vi "Arrow Drawing Utility.vi"(0 "LF Pod Setpoint":cluster{"Velocity":dbl, "Theta":dbl}, 5 "LB Pod Setpoint":cluster{"Velocity":dbl, "Theta":dbl}, 7 "RF Pod Setpoint":cluster{"Velocity":dbl, "Theta":dbl}, 9 "RB Pod Setpoint":cluster{"Velocity":dbl, "Theta":dbl}, 12 "cross products":T1, 13 "Translation":dbl[](array[numeric])) -> (4 "Pod Vectors":cluster{dbl[], dbl[]}[](array[cluster]), 6 "Translation Vectors":cluster{dbl[], dbl[]}, 8 "Rotation Vectors":cluster{dbl[], dbl[]})   [LabVIEW 2020]
uses:
  <vilib>/ptbypt/NI_PtbyPt.lvlib
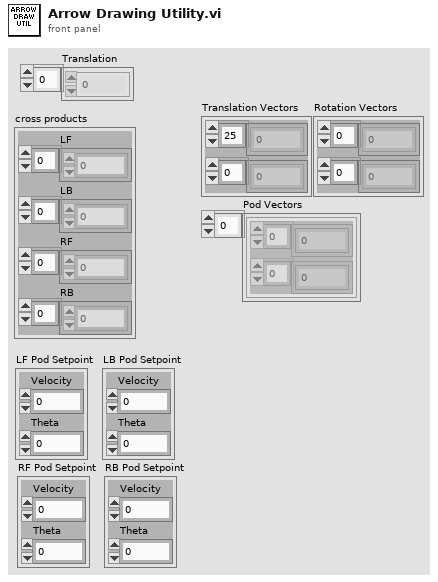
[diagram p1: front panel]
types:
  T1 = cluster{"LF":dbl[], "LB":dbl[], "RF":dbl[], "RB":dbl[]}
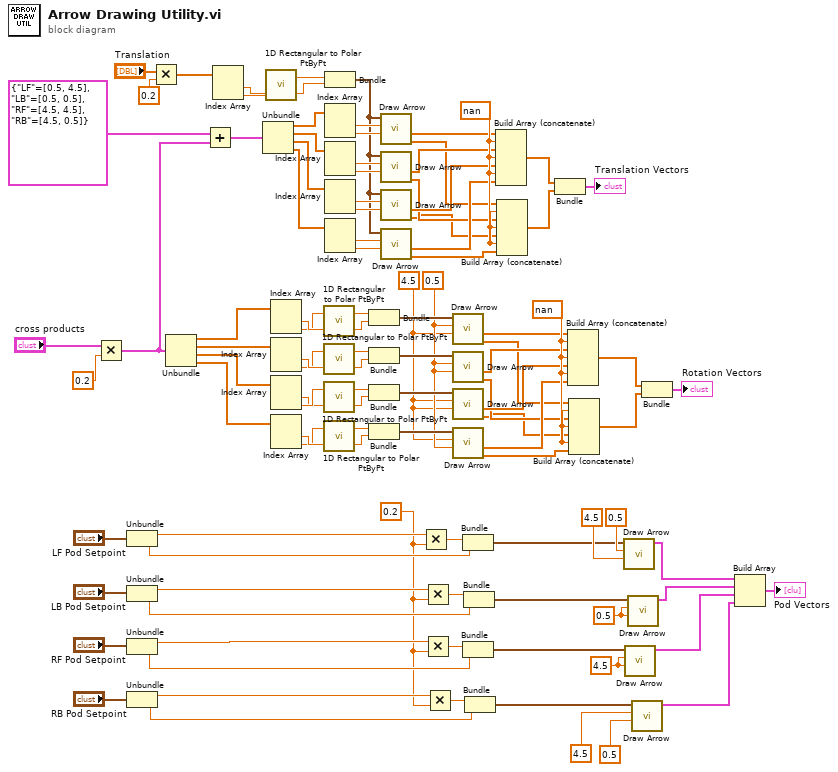
[diagram p0: block diagram]
diagram:
  w41 = nan ("Start Y")
  w54 = nan ("Start Y")
  w55 = 4.5 ("Start Y")
  w56 = 0.5 ("Start X")
  w81 = 0.2 ("y")
  w106 = 4.5 ("Start X")
  w107 = 0.5 ("Start X")
  n1 = Multiply(x="cross products", y=0.2) -> (x*y=w7:T1)
  n2 = Unbundle("LF Pod Setpoint") -> ("Velocity"=w97:dbl, "Theta"=w92:dbl)
  n3 = Unbundle("LB Pod Setpoint") -> ("Velocity"=w96:dbl, "Theta"=w88:dbl)
  n4 = Unbundle("RF Pod Setpoint") -> ("Velocity"=w95:dbl, "Theta"=w87:dbl)
  n5 = Unbundle("RB Pod Setpoint") -> ("Velocity"=w94:dbl, "Theta"=w86:dbl)
  n6 = Multiply(x="Translation", y=0.2) -> (x*y=w9:dbl[])
  n7 = Unbundle(w7) -> ("LF"=w80:dbl[], "LB"=w79:dbl[], "RF"=w78:dbl[], "RB"=w77:dbl[])
  n8 = Add(x=T1 {"LF"=[0.5, 4.5], "LB"=[0.5, 0.5], "RF"=[4.5, 4.5], "RB"=[4.5, 0.5]}, y=w7) -> (x+y=w42:T1)
  n9 = Index Array(array=w9) -> (element #1=w44:dbl, element #2=w43:dbl)  [unwired: 2 in]
  n10 = Unbundle(w42) -> ("LF"=w32:dbl[], "LB"=w31:dbl[], "RF"=w30:dbl[], "RB"=w29:dbl[])
  n11 = call <vilib>:"1D Rectangular to Polar PtByPt.vi"("y"=w44, "x"=w43) -> ("phase"=w19:dbl, "magnitude"=w20:dbl)
  n12 = Index Array(array=w80) -> (element #1=w76:dbl, element #2=w75:dbl)  [unwired: 2 in]
  n13 = Index Array(array=w79) -> (element #1=w74:dbl, element #2=w70:dbl)  [unwired: 2 in]
  n14 = Index Array(array=w78) -> (element #1=w71:dbl, element #2=w72:dbl)  [unwired: 2 in]
  n15 = Index Array(array=w77) -> (element #1=w73:dbl, element #2=w69:dbl)  [unwired: 2 in]
  n16 = call <vilib>:"1D Rectangular to Polar PtByPt.vi"("y"=w76, "x"=w75) -> ("phase"=w68:dbl, "magnitude"=w67:dbl)
  n17 = call <vilib>:"1D Rectangular to Polar PtByPt.vi"("y"=w74, "x"=w70) -> ("phase"=w63:dbl, "magnitude"=w64:dbl)
  n18 = call <vilib>:"1D Rectangular to Polar PtByPt.vi"("y"=w71, "x"=w72) -> ("phase"=w61:dbl, "magnitude"=w62:dbl)
  n19 = call <vilib>:"1D Rectangular to Polar PtByPt.vi"("y"=w73, "x"=w69) -> ("phase"=w57:dbl, "magnitude"=w58:dbl)
  n20 = Bundle("magnitude"=w20, "phase"=w19) -> (w18:cluster{"magnitude":dbl, "phase":dbl})  [unwired: 1 in]
  n21 = Index Array(array=w32) -> (element #1=w28:dbl, element #2=w27:dbl)  [unwired: 2 in]
  n22 = Index Array(array=w31) -> (element #1=w26:dbl, element #2=w25:dbl)  [unwired: 2 in]
  n23 = Index Array(array=w30) -> (element #1=w24:dbl, element #2=w23:dbl)  [unwired: 2 in]
  n24 = Index Array(array=w29) -> (element #1=w22:dbl, element #2=w21:dbl)  [unwired: 2 in]
  n25 = Bundle("magnitude"=w67, "phase"=w68) -> (w66:cluster{"magnitude":dbl, "phase":dbl})  [unwired: 1 in]
  n26 = Bundle("magnitude"=w64, "phase"=w63) -> (w65:cluster{"magnitude":dbl, "phase":dbl})  [unwired: 1 in]
  n27 = Bundle("magnitude"=w62, "phase"=w61) -> (w60:cluster{"magnitude":dbl, "phase":dbl})  [unwired: 1 in]
  n28 = Bundle("magnitude"=w58, "phase"=w57) -> (w59:cluster{"magnitude":dbl, "phase":dbl})  [unwired: 1 in]
  n29 = call "Draw Arrow.vi"("Start Y"=w27, "Start X"=w28, "Vector"=w18) -> ("Y"=w36:dbl[], "X"=w40:dbl[])  [unwired: 6 in, 1 out]
  n30 = call "Draw Arrow.vi"("Start Y"=w25, "Start X"=w26, "Vector"=w18) -> ("Y"=w35:dbl[], "X"=w39:dbl[])  [unwired: 6 in, 1 out]
  n31 = call "Draw Arrow.vi"("Start Y"=w23, "Start X"=w24, "Vector"=w18) -> ("Y"=w34:dbl[], "X"=w38:dbl[])  [unwired: 6 in, 1 out]
  n32 = call "Draw Arrow.vi"("Start Y"=w21, "Start X"=w22, "Vector"=w18) -> ("Y"=w33:dbl[], "X"=w37:dbl[])  [unwired: 6 in, 1 out]
  n33 = Multiply(x=w97, y=w81) -> (x*y=w93:dbl)
  n34 = Multiply(x=w96, y=w81) -> (x*y=w89:dbl)
  n35 = Multiply(x=w95, y=w81) -> (x*y=w91:dbl)
  n36 = Multiply(x=w94, y=w81) -> (x*y=w90:dbl)
  n37 = call "Draw Arrow.vi"("Start Y"=w55, "Start X"=w56, "Vector"=w66) -> ("Y"=w49:dbl[], "X"=w53:dbl[])  [unwired: 6 in, 1 out]
  n38 = call "Draw Arrow.vi"("Start Y"=w56, "Start X"=w56, "Vector"=w65) -> ("Y"=w48:dbl[], "X"=w52:dbl[])  [unwired: 6 in, 1 out]
  n39 = call "Draw Arrow.vi"("Start Y"=w55, "Start X"=w55, "Vector"=w60) -> ("Y"=w47:dbl[], "X"=w51:dbl[])  [unwired: 6 in, 1 out]
  n40 = call "Draw Arrow.vi"("Start Y"=w56, "Start X"=w55, "Vector"=w59) -> ("Y"=w46:dbl[], "X"=w50:dbl[])  [unwired: 6 in, 1 out]
  n41 = Bundle(w93, "Theta"=w92) -> (w85:cluster{dbl, "Theta":dbl})  [unwired: 1 in]
  n42 = Bundle(w91, "Theta"=w87) -> (w83:cluster{dbl, "Theta":dbl})  [unwired: 1 in]
  n43 = Bundle(w89, "Theta"=w88) -> (w84:cluster{dbl, "Theta":dbl})  [unwired: 1 in]
  n44 = Bundle(w90, "Theta"=w86) -> (w82:cluster{dbl, "Theta":dbl})  [unwired: 1 in]
  n45 = Build Array (concatenate)(w40, w41, w39, w41, w38, w41, w37) -> (w17:dbl[])
  n46 = Build Array (concatenate)(w36, w41, w35, w41, w34, w41, w33) -> (w16:dbl[])
  n47 = Bundle(w17, w16) -> (→"Translation Vectors":cluster{dbl[], dbl[]})  [unwired: 1 in]
  n48 = Build Array (concatenate)(w53, w54, w52, w54, w51, w54, w50) -> (w15:dbl[])
  n49 = Build Array (concatenate)(w49, w54, w48, w54, w47, w54, w46) -> (w14:dbl[])
  n50 = call "Draw Arrow.vi"("Start Y"=4.5, "Start X"=0.5, "Vector"=w85) -> ("Points"=w5:cluster{dbl[], dbl[]})  [unwired: 6 in, 2 out]
  n51 = call "Draw Arrow.vi"("Start Y"=w106, "Start X"=w106, "Vector"=w83) -> ("Points"=w3:cluster{dbl[], dbl[]})  [unwired: 6 in, 2 out]
  n52 = call "Draw Arrow.vi"("Start Y"=w107, "Start X"=w107, "Vector"=w84) -> ("Points"=w4:cluster{dbl[], dbl[]})  [unwired: 6 in, 2 out]
  n53 = call "Draw Arrow.vi"("Start Y"=0.5, "Start X"=4.5, "Vector"=w82) -> ("Points"=w2:cluster{dbl[], dbl[]})  [unwired: 6 in, 2 out]
  n54 = Bundle(w15, w14) -> (→"Rotation Vectors":cluster{dbl[], dbl[]})  [unwired: 1 in]
  n55 = Build Array(w5, w4, w3, w2) -> (→"Pod Vectors":cluster{dbl[], dbl[]}[])
